vi "Get AI Signal - Single.vi"(0 "reference in":refnum<class "AI.lvclass">, 3 "AI Channel Number (Zero Based)":i32, 4 "Zero Threshold":dbl, 5 "error in (no error)":errorcluster, 7 "Filter?":bool) -> (14 "reference out":refnum<class "AI.lvclass">, 15 "AI Channel Readings":dbl[](array[numeric]), 16 "AI Channel Sample Average":dbl, 17 "AI Channel Sample Standard Deviation":dbl, 18 "AI Channel Signal is Zero":bool, 19 "error out":errorcluster)   [LabVIEW 2017, in "AI.lvclass"]
uses:
  AI.lvclass
  <vilib>/Analysis/NI_AALBase.lvlib
panel:
  out "AI Channel Reading Chart":dbl[](graph)
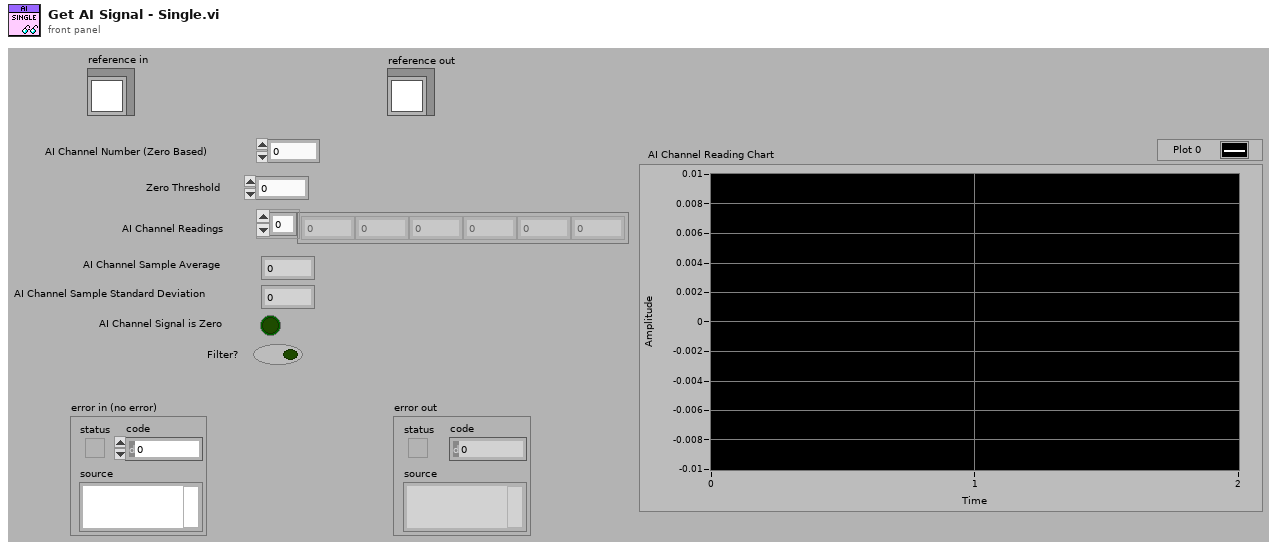
[diagram p1: front panel]
types:
  T1 = typedef "AI.lvclass/ObjectAttributes.ctl" = cluster{"AI Task":refnum<k21>, "AI On/Off Status":bool, "AI Sampling Rate (Samples/Seconds)":u32, "Number of AI Samples Per Channel":i32, "AI Voltage Range":u8, "AI Readings":dbl[][], "Number of AI Modules":i32, "Number of Total AI Channels":i32, "AI Module Names (NI-Max Name)":string[], "Number of Channels Per AI  Module":i32[], "AI VI Reference":refnum<vi>}
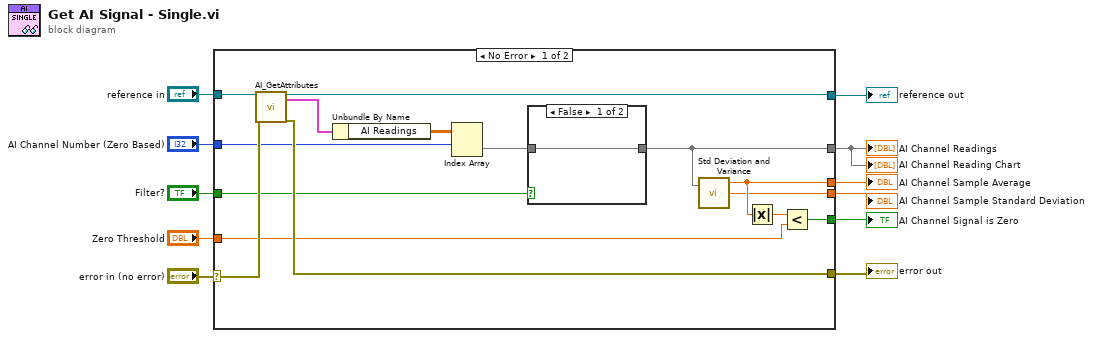
[diagram p0: block diagram]
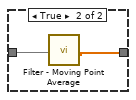
[diagram p2: hidden frame]
diagram:
  n1 = case shown="No Error" "error in (no error)" {
    selector: "error in (no error)" -> [w25 w31]
    tunnel: [w23 w31] -> w10
    tunnel: [w24 w30] -> w8
    tunnel: "reference in" -> [w26 w30]
    tunnel: "AI Channel Number (Zero Based)" -> [w22 _]
    tunnel: [w21 _] -> w4
    tunnel: [w20 _] -> w6
    tunnel: [w19 _] -> w5
    tunnel: [w13 _] -> w3
    tunnel: "Zero Threshold" -> [w15 _]
    tunnel: "Filter?" -> [w12 _]
    frame No Error {
      n2 = call "AI_GetAttributes.vi"("reference in"=w26, "error in (no error)"=w25) -> ("reference out"=w24:refnum<class "AI.lvclass">, "Data"=w16:T1, "error out"=w23:errorcluster)  [unwired: 14 in, 1 out]
      n3 = Unbundle By Name(w16) -> ("AI Readings"=w18:dbl[][])
      n4 = Index Array(array=w18, index (row)=w22) -> (element=w14:dbl[])  [unwired: 1 in]
      n5 = case shown="False" w12 {
        tunnel: w14 -> [w27 w29]
        tunnel: [w27 w28] -> w13
        frame False {
        }
        frame True {
          n6 = call "Filter - Moving Point Average.vi"("Analog Signal"=w29) -> ("Filtered Analog Signal"=w28:dbl[])  [unwired: 10 in]
        }
      }
      n7 = call <vilib>:"Std Deviation and Variance.vi"("X"=w13) -> ("mean"=w21:dbl, "standard deviation"=w19:dbl)  [unwired: 1 in, 1 out]
      n8 = Absolute Value(x=w21) -> (abs(x)=w17:dbl)
      n9 = Less?(x=w17, y=w15) -> (x < y?=w20:bool)
    }
    frame Error {
    }
  }
  "error out" <- w10
  "reference out" <- w8
  "AI Channel Readings" <- w3
  "AI Channel Signal is Zero" <- w6
  "AI Channel Sample Standard Deviation" <- w5
  "AI Channel Sample Average" <- w4
  "AI Channel Reading Chart" <- w3
